vi "calculator.vi"() -> ()   [LabVIEW 2021]
panel:
  in  "stop":bool
  out "Time Stamp":timestamp
  in  "operation":string(combo)
  out "Answer":dbl
  in  "Operand2":dbl
  in  "Operand1":dbl
  out "Cal display":string
  in  "Numeric 2":i32
  out "System Time (second)":i32
  out "cal display2":string
  in  "(":bool
  in  ")":bool
  in  "CE":bool
  in  "C":bool
  in  "Backspace":bool
  in  "√":bool
  in  "1/x":bool
  in  "+/-":bool
  in  "Div":bool
  in  "Mul":bool
  in  "Add":bool
  in  "Sub":bool
  in  "=":bool
  in  ".":bool
  in  "4":bool
  in  "0":bool
  in  "9":bool
  in  "8":bool
  in  "7":bool
  in  "6":bool
  in  "5":bool
  in  "3":bool
  in  "2":bool
  in  "1":bool
  # "Calculator"
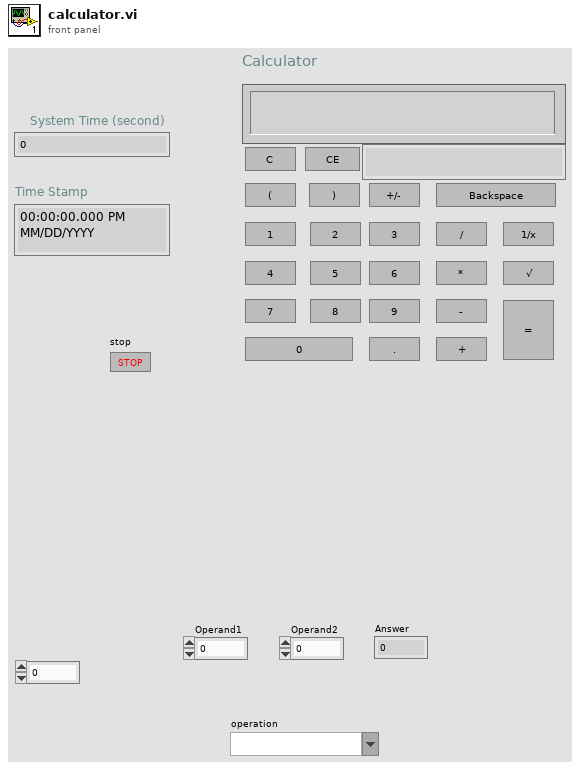
[diagram p1: front panel]
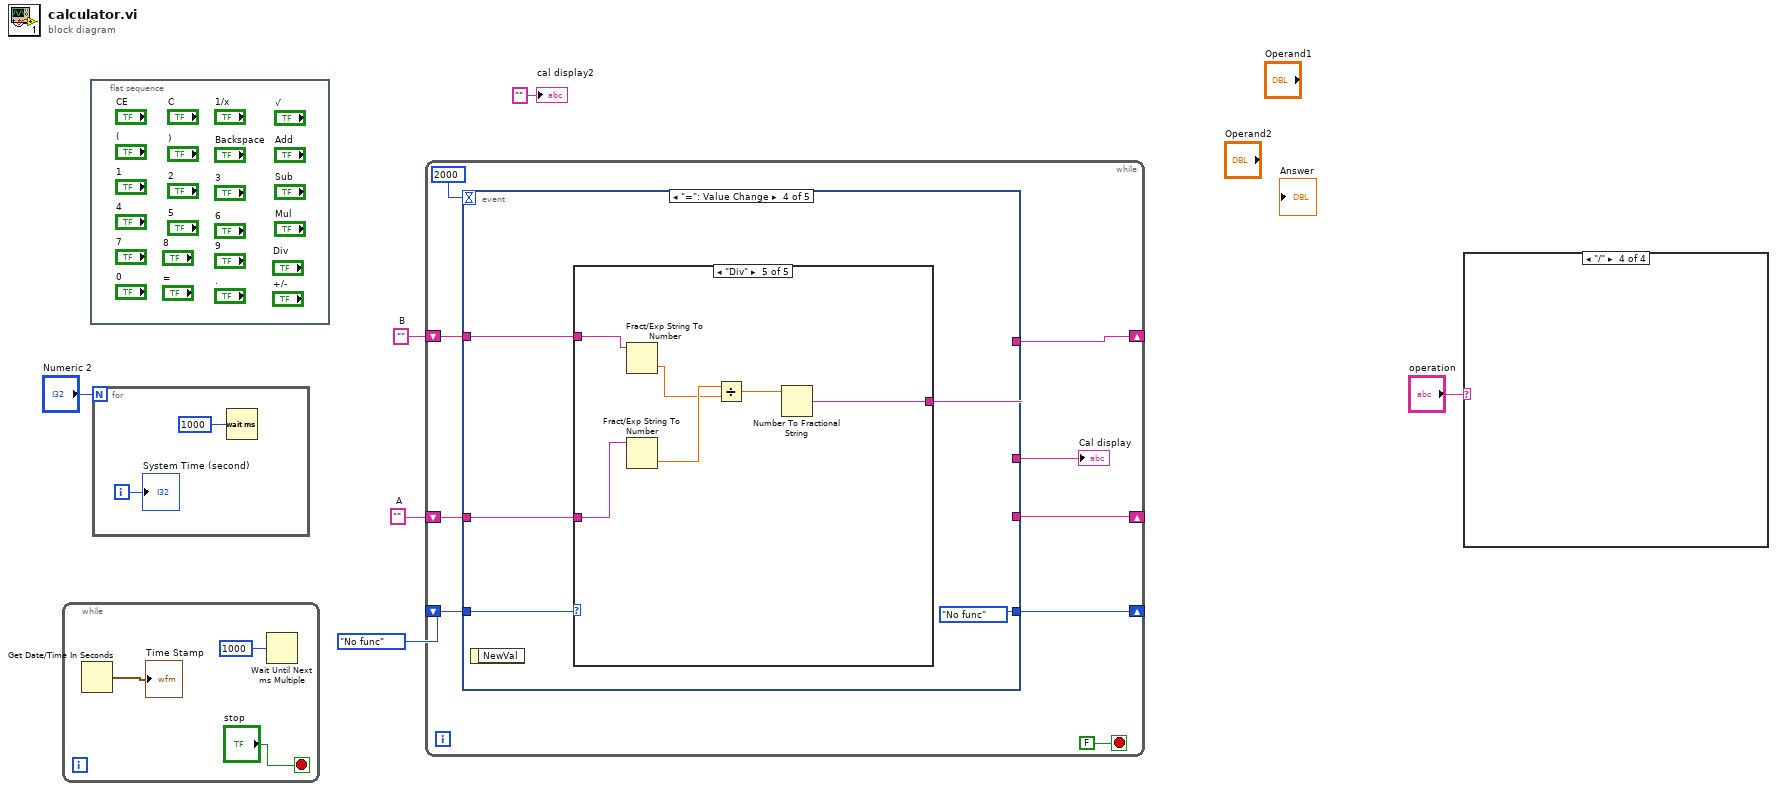
[diagram p0: block diagram]
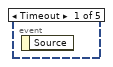
[diagram p5: hidden frame]
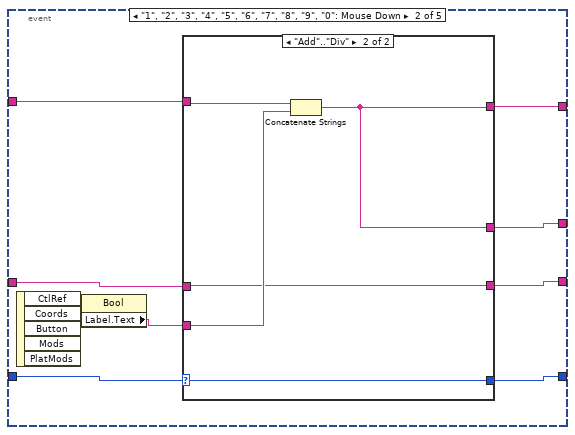
[diagram p6: hidden frame]
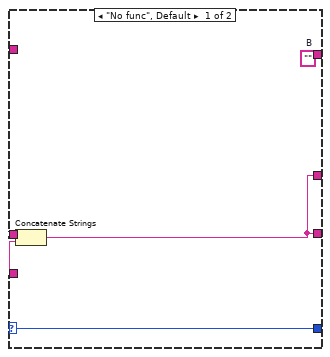
[diagram p7: hidden frame]
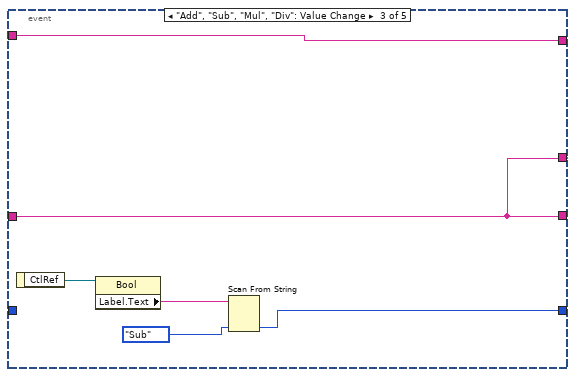
[diagram p8: hidden frame]
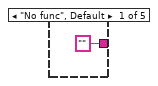
[diagram p9: hidden frame]
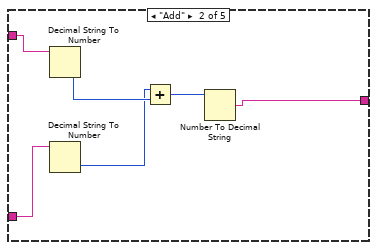
[diagram p10: hidden frame]
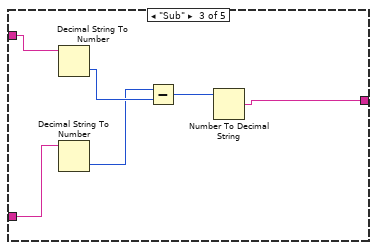
[diagram p11: hidden frame]
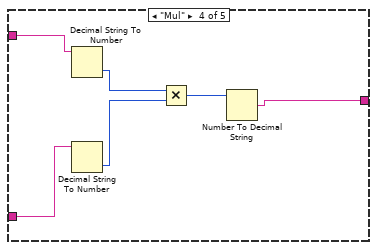
[diagram p12: hidden frame]
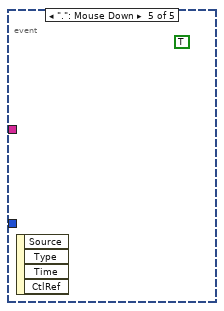
[diagram p13: hidden frame]
diagram:
  w6 = ""  # A
  w5 = ""  # B
  n1 = while {
    stop <- "stop" stop-if-true
    n2 = Get Date/Time In Seconds() -> (seconds since 1Jan1904=→"Time Stamp":timestamp)
    n3 = Wait Until Next ms Multiple(millisecond multiple=1000) -> ()  [unwired: 1 out]
  }
  n4 = flat-sequence {
    frame #0 {
    }
  }
  n5 = for {
    N: "Numeric 2" -> [_]
    i -> [w11]
    n6 = Wait (ms)(milliseconds to wait=u32 1000 ("millisecond timer value")) -> ()  [unwired: 1 out]
    "System Time (second)" <- w11
  }
  n7 = while {
    shift-right: [w15] -> _
    shift-left: w5 -> [w19]
    shift-right: [w16] -> _
    shift-left: w6 -> [w20]
    shift-right: [w17] -> _
    shift-left: enum16{"No func", "Add", "Sub", "Mul", "Div"}."No func" -> [w18]
    stop <- FALSE stop-if-true
    n8 = event shown="[3] \"=\": Value Change" {
      selector: _ -> [_ _ _ _ _]
      dyn-events: _ -> [_ _ _ _ _]
      timeout: 2000 -> [_ _ _ _ _]
      tunnel: w20 -> [_ w27 w41 w48 _]
      tunnel: w19 -> [_ w24 w45 w47 _]
      tunnel: w18 -> [_ w28 _ w49 _]
      tunnel: [_ w21 w42 enum16{"No func", "Add", "Sub", "Mul", "Div"}."No func" _] -> w17
      tunnel: [_ w25 w41 _ _] -> w16
      tunnel: [_ w23 w45 _ _] -> w15
      tunnel: [_ w22 w41 w50 _] -> w14
      event Timeout {
        n9 = event-data() -> ()  [unwired: 1 in, 1 out]
      }
      event "1", "2", "3", "4", "5", "6", "7", "8", "9", "0": Mouse Down {
        n10 = event-data() -> ("CtlRef"=w29:refnum<vi>)  [unwired: 1 in, 4 out]
        n11 = property class="Bool"(reference=w29) -> ("Label.Text"=w26:string)  [unwired: 1 in, 2 out]
        n12 = case shown="\"Add\"..\"Div\"" w28 {
          selector: w28 -> [w30 w35]
          tunnel: w27 -> [w34 w37]
          tunnel: w26 -> [w33 w38]
          tunnel: [w31 w37] -> w25
          tunnel: w24 -> [_ w39]
          tunnel: [w32 w36] -> w23
          tunnel: [w31 w36] -> w22
          tunnel: [w30 w35] -> w21
          frame "No func", Default {
            w32 = ""  # B
            n13 = Concatenate Strings(w34, w33) -> (w31:string)
          }
          frame "Add".."Div" {
            n14 = Concatenate Strings(w39, w38) -> (w36:string)
          }
        }
      }
      event "Add", "Sub", "Mul", "Div": Value Change {
        n15 = event-data() -> ("CtlRef"=w43:refnum<vi>)  [unwired: 1 in]
        n16 = property class="Bool"(reference=w43) -> ("Label.Text"=w44:string)  [unwired: 1 in, 2 out]
        n17 = Scan From String "Scan From String"(input string=w44, default 1=enum16{"No func", "Add", "Sub", "Mul", "Div"}."Sub") -> (output 1=w42:enum16{"No func", "Add", "Sub", "Mul", "Div"})  [unwired: 3 in, 3 out]
      }
      event "=": Value Change {
        n18 = event-data() -> ()  [unwired: 1 in, 1 out]
        n19 = case shown="\"Div\"" w49 {
          tunnel: ["" w56 w58 w64 w75] -> w50
          tunnel: w48 -> [_ w55 w59 w65 w72]
          tunnel: w47 -> [_ w57 w60 w66 w71]
          frame "No func", Default {
          }
          frame "Add" {
            n20 = Decimal String To Number(string=w57) -> (number=w54:i32)  [unwired: 2 in, 1 out]
            n21 = Decimal String To Number(string=w55) -> (number=w53:i32)  [unwired: 2 in, 1 out]
            n22 = Add(x=w53, y=w54) -> (x+y=w52:i32)
            n23 = Number To Decimal String(number=w52) -> (decimal integer string=w56:string)  [unwired: 1 in]
          }
          frame "Sub" {
            n24 = Decimal String To Number(string=w60) -> (number=w63:i32)  [unwired: 2 in, 1 out]
            n25 = Decimal String To Number(string=w59) -> (number=w62:i32)  [unwired: 2 in, 1 out]
            n26 = Subtract(x=w62, y=w63) -> (x-y=w61:i32)
            n27 = Number To Decimal String(number=w61) -> (decimal integer string=w58:string)  [unwired: 1 in]
          }
          frame "Mul" {
            n28 = Decimal String To Number(string=w66) -> (number=w69:i32)  [unwired: 2 in, 1 out]
            n29 = Decimal String To Number(string=w65) -> (number=w68:i32)  [unwired: 2 in, 1 out]
            n30 = Multiply(x=w69, y=w68) -> (x*y=w67:i32)
            n31 = Number To Decimal String(number=w67) -> (decimal integer string=w64:string)  [unwired: 1 in]
          }
          frame "Div" {
            n32 = Fract/Exp String To Number(string=w71) -> (number=w73:dbl)  [unwired: 3 in, 1 out]
            n33 = Fract/Exp String To Number(string=w72) -> (number=w74:dbl)  [unwired: 3 in, 1 out]
            n34 = Divide(x=w74, y=w73) -> (x/y=w70:dbl)
            n35 = Number To Fractional String(number=w70) -> (F-format string=w75:string)  [unwired: 3 in]
          }
        }
      }
      event ".": Mouse Down {
        (unwired) TRUE
        n36 = event-data() -> ()  [unwired: 1 in, 4 out]
      }
    }
    "Cal display" <- w14
  }
  n37 = case shown="\"/\"" "operation" {
    frame "*", Default {
    }
    frame "+" {
    }
    frame "-" {
    }
    frame "/" {
    }
  }
  "cal display2" <- "" ("cal display2")
